vi "Get vacuum.vi"(8 "error in (no error)":errorcluster, 11 "Pressure Control in":refnum<class "Pressure Control.lvclass">) -> (0 "error out":errorcluster, 2 "Vacuum?":bool, 3 "Pressure Control out":refnum<class "Pressure Control.lvclass">)   [LabVIEW 2011, in "Pressure Control.lvclass"]
uses:
  Pressure Control.lvclass
  Pressure Control.lvclass/Pressure Control.ctl
  TTL/TTL.lvclass
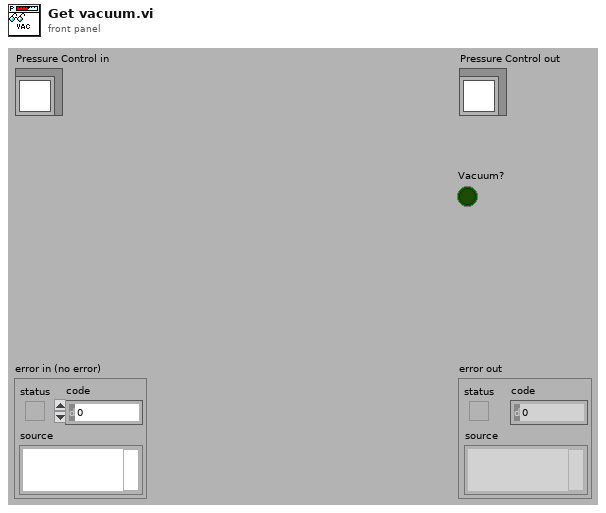
[diagram p1: front panel]
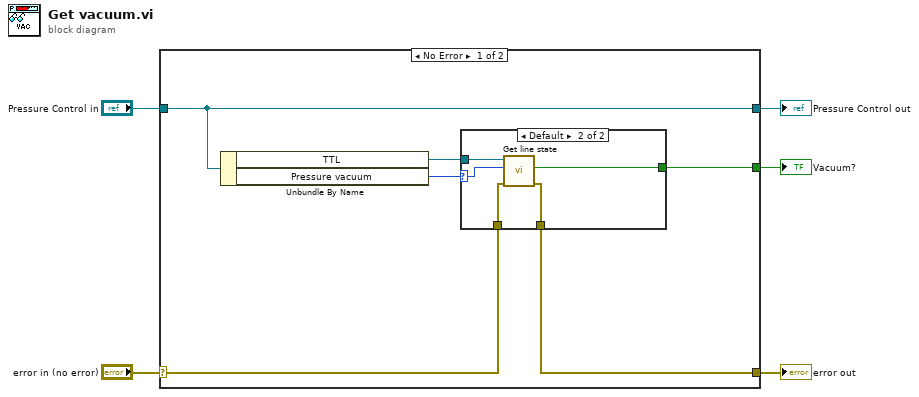
[diagram p0: block diagram]
diagram:
  n1 = case shown="No Error" "error in (no error)" {
    selector: "error in (no error)" -> [w8 w19]
    tunnel: [w7 w19] -> w4
    tunnel: [w11 w18] -> w2
    tunnel: "Pressure Control in" -> [w11 w18]
    tunnel: [w6 _] -> w1
    frame No Error {
      n2 = Unbundle By Name(w11) -> ("TTL"=w9:refnum<class "TTL.lvclass">, "Pressure vacuum"=w10:i32)
      n3 = case shown="Default" w10 {
        selector: w10 -> [_ w16]
        tunnel: w9 -> [_ w17]
        tunnel: w8 -> [w12 w15]
        tunnel: [w12 w14] -> w7
        tunnel: [_ w13] -> w6
        frame -1 {
          # "No \"vacuum\" line was defined\nin the hardware config"
        }
        frame Default {
          n4 = call "Get line state.vi"("error in (no error)"=w15, "Line number"=w16, "TTL in"=w17) -> ("error out"=w14:errorcluster, "Line state"=w13:bool)  [unwired: 6 in, 1 out]
        }
      }
    }
    frame Error {
    }
  }
  "error out" <- w4
  "Pressure Control out" <- w2
  "Vacuum?" <- w1
